vi "ZPL Transient Store.vi"(6 "Settle (1 mS)":u32=1, 8 "error":errorcluster, 9 "Memory SAVE":u16(ring)=3 items=["1", "2", "3", "4"], 10 "Save Mode":u16(ring)=1 items=["LIST", "WAVE"], 11 "VISA":refnum<visa-resource-name>) -> (0 "error out":errorcluster, 3 "VISA out":refnum<visa-resource-name>)   [LabVIEW 2015]
doc: "This command save under specifies number <1..4> the last selected LIST/WAVE type (voltage or/and current) , type values and time values from volatile memory\n\nLIST and WAVE store in cell are same. So when data stored in cell <n> in WAVE it overwrite on data stored in LIST with same number"
panel:
  # "Lambda ZPLUS \n Serial Port\n  DC Power Supplies"
  # "Command STORE LIST/WAVE values"
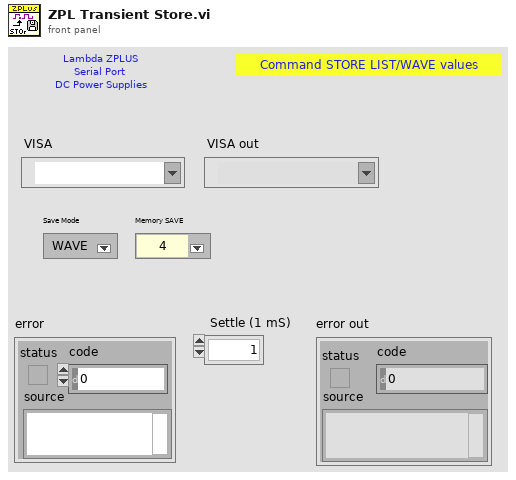
[diagram p1: front panel]
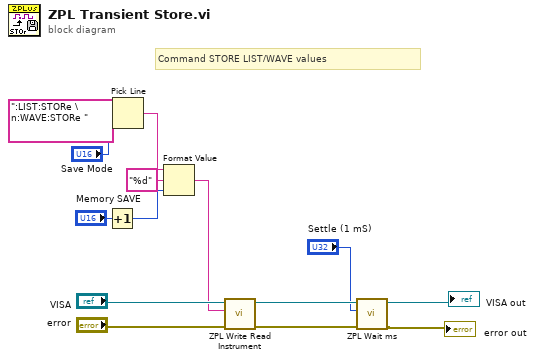
[diagram p0: block diagram]
diagram:
  # "Command STORE LIST/WAVE values"
  n1 = Increment(x="Memory SAVE") -> (x+1=w4:u16)
  n2 = Pick Line(multi-line string=":LIST:STORe \n:WAVE:STORe ", line index="Save Mode") -> (output string=w1:string)  [unwired: 1 in]
  n3 = Format Value(string ("")=w1, format string="%d", value (0)=w4) -> (output string=w5:string)
  n4 = call "ZPL Write Read Instrument.vi"("error in"="error", "Write Command/Query SCPI"=w5, "VISA"="VISA") -> ("error out"=w11:errorcluster, "VISA  out"=w12:refnum<visa-resource-name>)  [unwired: 6 in, 1 out]
  n5 = call "ZPL Wait ms.vi"("error"=w11, "Delay (1 mS)"="Settle (1 mS)", "VISA"=w12) -> ("error out"=→"error out":errorcluster, "VISA out"=→"VISA out":refnum<visa-resource-name>)  [unwired: 7 in]
